vi "safe state stop and close.vi"(8 "error in":errorcluster, 11 "message queue in":T1) -> (0 "error out":errorcluster, 3 "message queue out":T1)   [LabVIEW 2013, in "DCAF message service.lvlib"]
doc: "Use this VI to stop and close all engines currently running on the target."
uses:
  DCAF message service.lvlib
  <vilib>/NI/AMC/Message Queue.ctl
  <vilib>/NI/AMC/Message.ctl
  <vilib>/NI/Tools/Keyed Array/KeyedArray.ctl
  command commands to rtexe process.ctl
  <vilib>/NI/Tools/Keyed Array/Tools_KeyedArray.lvlib
  <vilib>/NI/AMC/AMC.lvlib
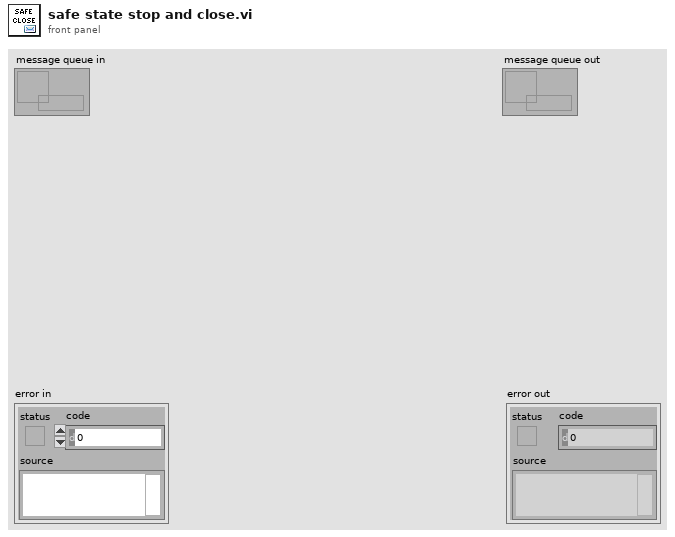
[diagram p1: front panel]
types:
  T1 = typedef "AMC.lvlib/Message Queue.ctl" = refnum<queue>
  T2 = typedef "DCAF message service.lvlib/command commands to rtexe process.ctl" = enum16{"Initialize", "Add Search Paths", "Load from File", "Unload File", "Open All Engines", "Open Single Engine", "Initialize All Engines", "Initialize Single Engine", "Start All", "Start Single", "Pause All", "Pause Single", "Stop All", "Stop Single", "Close All", "Close Single", "Set Safe State All", "Set Safe State Single", "Get Status", "Exit", "Error", "Load Bitfile", "Unload Bitfile", "Clear Faults Single", "Clear Faults All"}
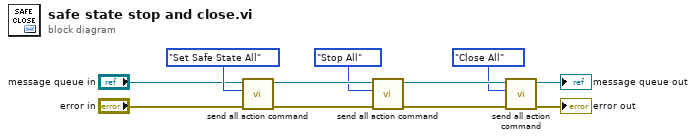
[diagram p0: block diagram]
diagram:
  n1 = call "send all action command.vi"("error in"="error in", "commands"=command_commands_to_rtexe_process."Set Safe State All", "message queue in"="message queue in") -> ("error out"=w9:errorcluster, "message queue out"=w8:T1)  [unwired: 7 in]
  n2 = call "send all action command.vi"("error in"=w9, "commands"=command_commands_to_rtexe_process."Stop All", "message queue in"=w8) -> ("error out"=w11:errorcluster, "message queue out"=w10:T1)  [unwired: 7 in]
  n3 = call "send all action command.vi"("error in"=w11, "commands"=command_commands_to_rtexe_process."Close All", "message queue in"=w10) -> ("error out"=→"error out":errorcluster, "message queue out"=→"message queue out":T1)  [unwired: 7 in]
